vi "WaitOnReady.vi"(0 "AddressSpace in":refnum<class "AddressSpace.lvclass">) -> (4 "AddressSpace out":refnum<class "AddressSpace.lvclass">)   [LabVIEW 2017, in "BuckBoost.lvlib"]
uses:
  BuckBoost.lvlib
  AddressSpace.lvclass
  <vilib>/rvi/Emulation/niFpgaGetClockAttributes.vi
  <vilib>/rvi/Emulation/niFpgaSctlEmulationGetInTimedLoop.vi
  <vilib>/rvi/Emulation/niFpgaEmulationReportErrorSimple.vi
  <vilib>/rvi/Emulation/niFpgaCriticalErrorInLSC.vi
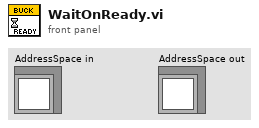
[diagram p1: front panel]
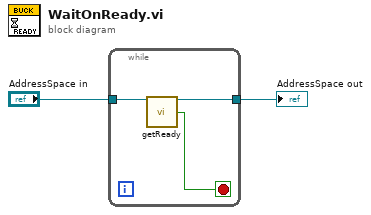
[diagram p0: block diagram]
diagram:
  n1 = while {
    tunnel: "AddressSpace in" -> [w5]
    tunnel: [w3] -> w1
    stop <- w4 stop-if-true
    n2 = call "getReady.vi"("AddressSpace in"=w5) -> ("AddressSpace out"=w3:refnum<class "AddressSpace.lvclass">, "ready"=w4:bool)  [unwired: 13 in]
  }
  "AddressSpace out" <- w1
